vi "Write Input Graph.vi"(8 "error in (no error)":errorcluster, 10 "Input Graph":refnum<vi>, 11 "AbstractExtractor1D in":refnum<class "AbstractExtractor1D.lvclass">) -> (0 "error out":errorcluster, 3 "AbstractExtractor1D out":refnum<class "AbstractExtractor1D.lvclass">)   [LabVIEW 2014]
uses:
  AbstractExtractor1D.lvclass
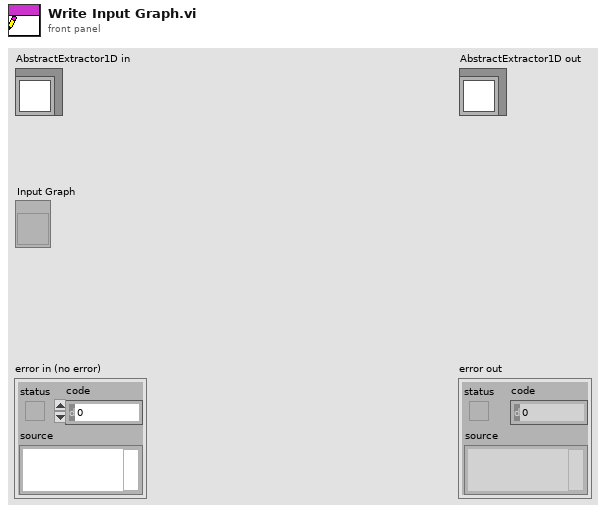
[diagram p1: front panel]
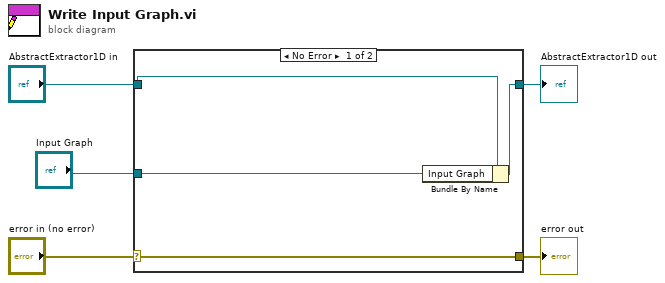
[diagram p0: block diagram]
diagram:
  n1 = case shown="No Error" "error in (no error)" {
    selector: "error in (no error)" -> [w9 w10]
    tunnel: [w9 w10] -> w4
    tunnel: [w7 w11] -> w2
    tunnel: "AbstractExtractor1D in" -> [w8 w11]
    tunnel: "Input Graph" -> [w6 _]
    frame No Error {
      n2 = Bundle By Name(cluster=w8, "Input Graph"=w6) -> (w7:refnum<class "AbstractExtractor1D.lvclass">)
    }
    frame Error {
    }
  }
  "error out" <- w4
  "AbstractExtractor1D out" <- w2
